vi "Write Samples per read.vi"(8 "error in (no error)":errorcluster, 10 "Samples per read":i32=1024, 11 "RP Transceiver in":refnum<class "RP Transceiver.lvclass">) -> (0 "error out":errorcluster, 3 "RP Transceiver out":refnum<class "RP Transceiver.lvclass">)   [LabVIEW 2015, in "RP Transceiver.lvclass"]
uses:
  RP Transceiver.lvclass
  RP Transceiver.lvclass/RP Transceiver.ctl
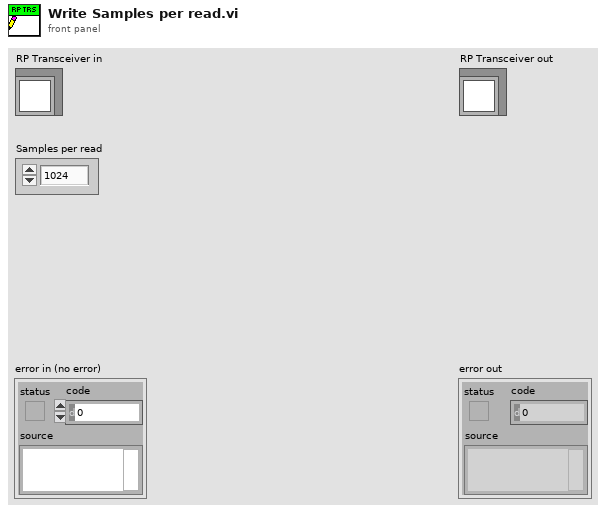
[diagram p1: front panel]
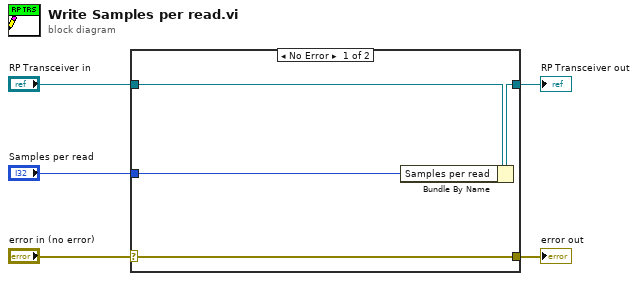
[diagram p0: block diagram]
diagram:
  n1 = case shown="No Error" "error in (no error)" {
    selector: "error in (no error)" -> [w9 w10]
    tunnel: [w9 w10] -> w4
    tunnel: [w7 w11] -> w2
    tunnel: "RP Transceiver in" -> [w8 w11]
    tunnel: "Samples per read" -> [w6 _]
    frame No Error {
      n2 = Bundle By Name(cluster=w8, "Samples per read"=w6) -> (w7:refnum<class "RP Transceiver.lvclass">)
    }
    frame Error {
    }
  }
  "error out" <- w4
  "RP Transceiver out" <- w2
